vi "Positioning.vi"(8 "error in (no error)":errorcluster, 9 "type":enum16{"Absolute (G90)", "Relative (G91)"}(ring)=enum."Relative (G91)", 11 "VISA resource name":refnum<visa-resource-name>) -> (0 "error out":errorcluster, 3 "VISA resource name out":refnum<visa-resource-name>)   [LabVIEW 2023, in "Marlin Instrument Driver.lvlib"]
doc: "Returns the current state of the configured X, Y, Z endstops. Takes into account any 'inverted endstop' settings, so one can confirm that the machine is interpreting the endstops correctly."
uses:
  Marlin Instrument Driver.lvlib
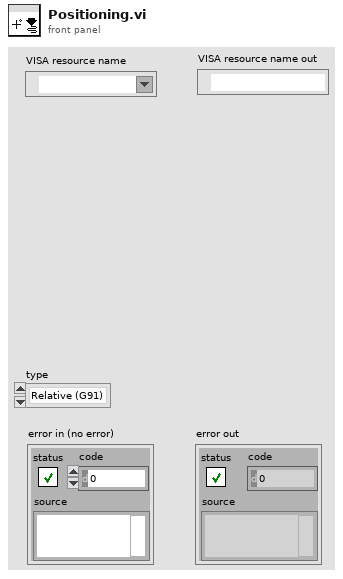
[diagram p1: front panel]
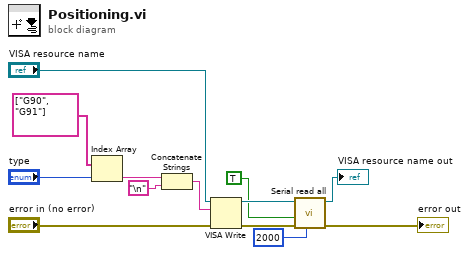
[diagram p0: block diagram]
diagram:
  n1 = Index Array(array=string[] ["G90", "G91"], index="type") -> (element=w1:string)
  n2 = Concatenate Strings(w1, "\n") -> (w2:string)
  n3 = VISA Write(VISA resource name="VISA resource name", write buffer=w2, error in (no error)="error in (no error)") -> (VISA resource name out=w10:refnum<visa-resource-name>, error out=w11:errorcluster)  [unwired: 1 out]
  n4 = call "Serial read all.vi"("timeout (10000ms)"=u32 2000, "error in (no error)"=w11, "Wait for OK"=TRUE, "VISA Refnum in"=w10) -> ("error out"=→"error out":errorcluster, "VISA Refnum out"=→"VISA resource name out":refnum<visa-resource-name>)  [unwired: 4 in, 2 out]
